vi "Get Platform Name.vi"(8 "error in (no error)":errorcluster, 11 "Device in":refnum<class "Device.lvclass">) -> (0 "error out":errorcluster, 2 "Platform Name":string, 3 "Device out":refnum<class "Device.lvclass">)   [LabVIEW 2020, in "PicoG-Core.lvlib" / "Device.lvclass"]
uses:
  Device.lvclass
  Device.lvclass/Device.ctl
  DeployPlatform/DeployPlatform.lvclass
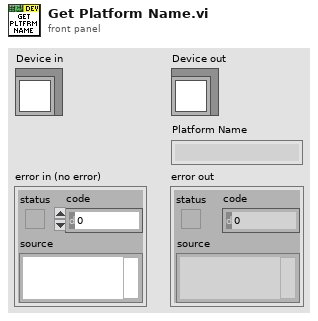
[diagram p1: front panel]
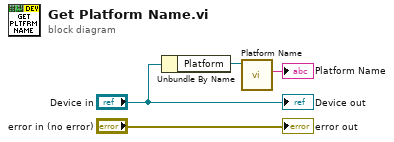
[diagram p0: block diagram]
diagram:
  n1 = Unbundle By Name("Device in") -> ("Platform"=w2:refnum<class "DeployPlatform.lvclass">)
  n2 = call-dynamic "Platform Name.vi"("DeployTarget in"=w2) -> ("Platform Name"=→"Platform Name":string)  [unwired: 8 in, 2 out]
  "error out" <- "error in (no error)"
  "Device out" <- "Device in"
